vi "BB_CameraMJPG-StreamerRead.vi"(0 "Refnum in":T1, 1 "Operation":enum16{"Read", "Reopen", "Close"}(ring), 2 "remote port or service name":u16=5800, 5 "address":string, 7 "fps":i32=30, 9 "millisecond timer value in":u32, 11 "error in (no error)":errorcluster, 12 "Numeric in":i32) -> (4 "Refnum out":T1, 6 "Numeric 3":i32, 8 "Numeric out":i32, 10 "millisecond timer value out":u32, 15 "error out":errorcluster)   [LabVIEW 2015]
uses:
  <vilib>/vision/Image Controls.llb/IMAQ Image.ctl
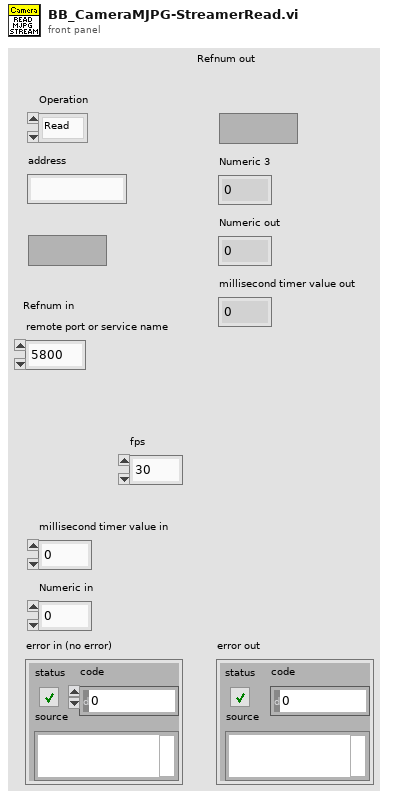
[diagram p1: front panel]
types:
  T1 = typedef "IMAQ Image.ctl" = refnum<image>
  T2 = enum16{"Standard", "Buffered", "CRLF", "Immediate"}
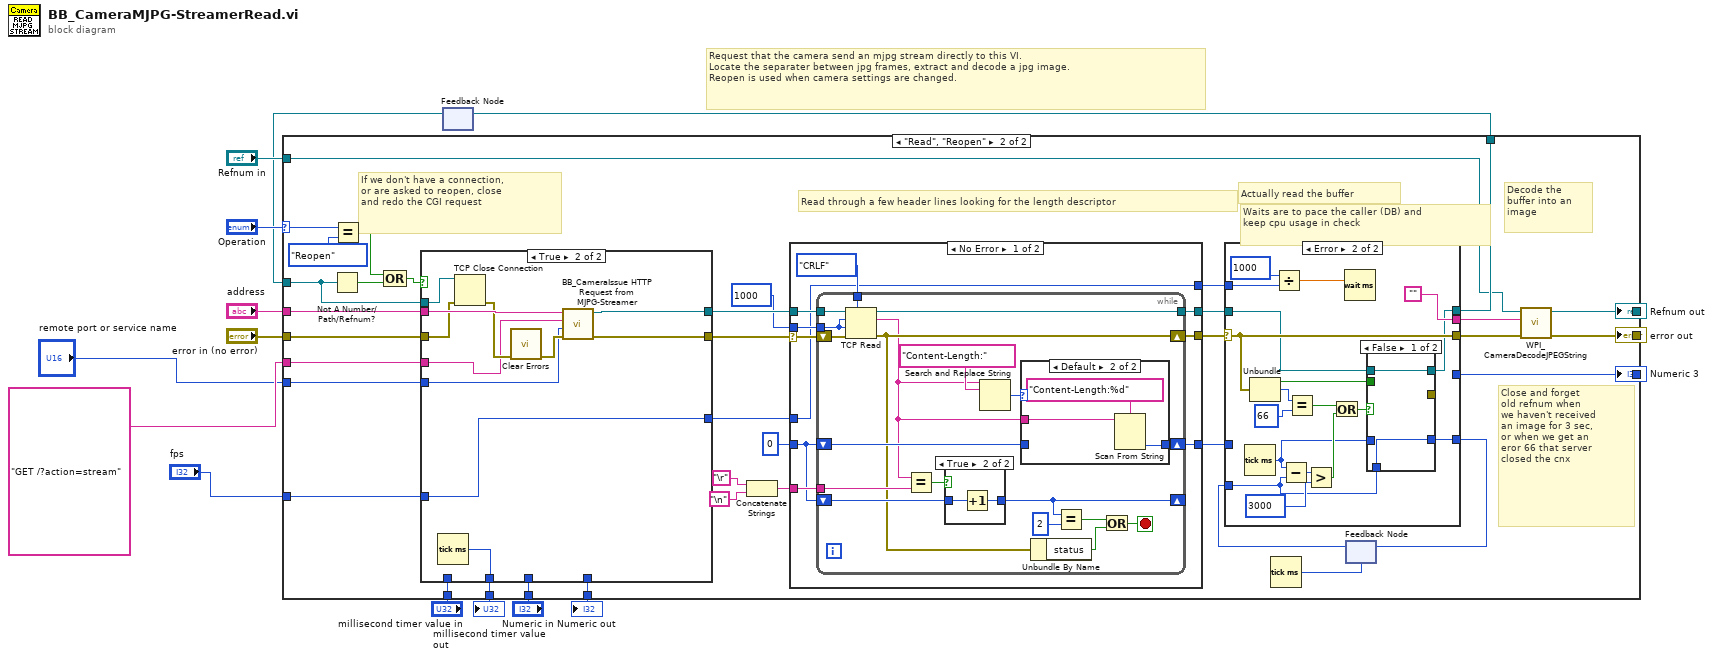
[diagram p0: block diagram]
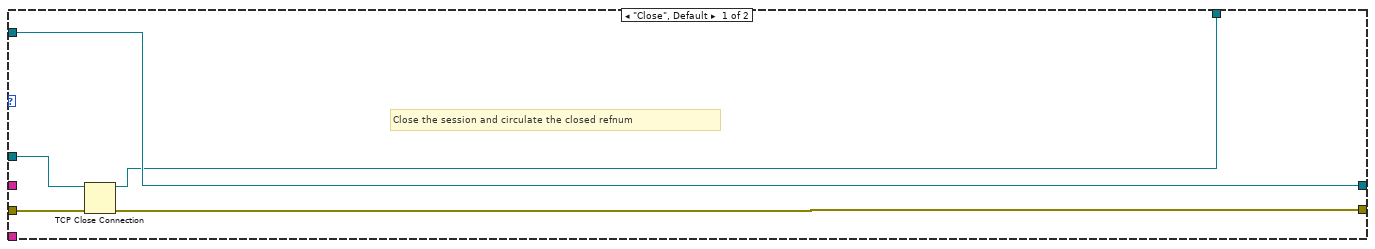
[diagram p2: hidden frame]
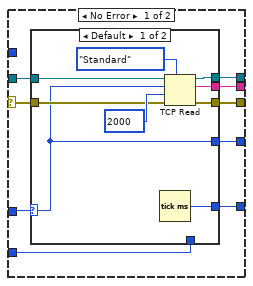
[diagram p4: hidden frame]
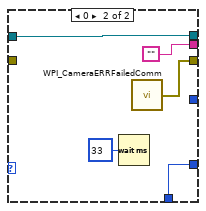
[diagram p5: hidden frame]
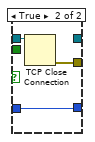
[diagram p6: hidden frame]
diagram:
  # "Request that the camera send an mjpg stream directly to this VI.\nLocate the separater between jpg frames, extract and decode a jpg image.\nReopen is used when camera settings are changed."
  n1 = feedback #1() -> (w9:refnum<k5>)  [unwired: 1 out]
  n2 = case shown="\"Read\", \"Reopen\"" "Operation" {
    selector: "Operation" -> [_ w38]
    tunnel: "error in (no error)" -> [w20 w49]
    tunnel: "address" -> [_ w48]
    tunnel: [w17 w47] -> w6
    tunnel: "GET /?action=stream" -> [_ w46]
    tunnel: [w18 w43] -> w7
    tunnel: [w19 w41] -> w8
    tunnel: w9 -> [w21 w39]
    tunnel: "Refnum in" -> [w18 w37]
    tunnel: [_ w33] -> w12
    tunnel: "Numeric in" -> [_ w32]
    tunnel: [_ w31] -> w14
    tunnel: "millisecond timer value in" -> [_ w30]
    tunnel: [_ w29] -> w16
    tunnel: "fps" -> [_ w23]
    tunnel: "remote port or service name" -> [_ w22]
    frame "Close", Default {
      # "Close the session and circulate the closed refnum"
      n3 = TCP Close Connection(connection ID=w21, error in (no error)=w20) -> (connection ID out=w17:refnum<k5>, error out=w19:errorcluster)  [unwired: 1 out]
    }
    frame "Read", "Reopen" {
      # "Waits are to pace the caller (DB) and\nkeep cpu usage in check"
      # "Close and forget\nold refnum when\nwe haven't received\nan image for 3 sec,\nor when we get an\neror 66 that server\nclosed the cnx"
      # "Decode the buffer into an image"
      # "Actually read the buffer"
      # "Read through a few header lines looking for the length descriptor"
      # "If we don't have a connection,\nor are asked to reopen, close\nand redo the CGI request"
      n4 = Not A Number/Path/Refnum?(number/path/refnum=w39) -> (NaN/Path/Refnum?=w27:bool)
      n5 = Equal?(x=w38, y=enum16{"Read", "Reopen", "Close"}."Reopen" ("Operation")) -> (x = y?=w28:bool)
      n6 = Compound Arithmetic op=OR(w28, w27) -> (w26:bool)
      n7 = case shown="True" w26 {
        tunnel: [w62 w72] -> w53
        tunnel: [w63 w73] -> w52
        tunnel: w49 -> [w62 w70]
        tunnel: w48 -> [_ w74]
        tunnel: w39 -> [w63 w71]
        tunnel: w46 -> [_ w66]
        tunnel: w32 -> [w61 _]
        tunnel: [w61 _] -> w31
        tunnel: w30 -> [w60 _]
        tunnel: [w60 w67] -> w29
        tunnel: [w59 w65] -> w24
        tunnel: w23 -> [w59 w65]
        tunnel: w22 -> [_ w64]
        frame False {
        }
        frame True {
          n8 = Tick Count (ms)() -> (millisecond timer value=w67:u32)
          n9 = TCP Close Connection(connection ID=w71, error in (no error)=w70) -> (error out=w69:errorcluster)  [unwired: 2 out]
          n10 = call <vilib>:"Clear Errors.vi"("error in (no error)"=w69) -> ("error out"=w68:errorcluster)  [unwired: 1 in, 5 out]
          n11 = call "BB_CameraIssue HTTP Request from MJPG-Streamer.vi"("error in (no error)"=w68, "remote port or service name"=w64, "Request"=w66, "address"=w74) -> ("error out"=w72:errorcluster, "connection ID (dup)"=w73:refnum<k5>)  [unwired: 6 out]
        }
      }
      n12 = Concatenate Strings("\r", "\n") -> (w56:string)
      n13 = case shown="No Error" w53 {
        selector: w53 -> [w123 w159]
        tunnel: [w130 w159] -> w50
        tunnel: [w129 w158] -> w55
        tunnel: [w128 w160] -> w54
        tunnel: w56 -> [w127 _]
        tunnel: w52 -> [w125 w160]
        tunnel: 1000 ("bytes to read") -> [w124 _]
        tunnel: 0 -> [w122 w158]
        tunnel: [w121 w157] -> w25
        tunnel: w24 -> [w121 w157]
        frame No Error {
          n14 = while {
            tunnel: w125 -> [w149]
            tunnel: [w148] -> w128
            shift-right: [w147] -> w129
            shift-left: w122 -> [w146]
            shift-right: [w143] -> _
            shift-left: w122 -> [w144]
            tunnel: w127 -> [w141]
            tunnel: w124 -> [w131]
            tunnel: T2."CRLF" ("mode (standard)") -> [w140]
            shift-right: [w138] -> w130
            shift-left: w123 -> [w139]
            stop <- w137 stop-if-true
            n15 = TCP Read(connection ID=w149, bytes to read=w131, error in (no error)=w139, 7:w140, 9:w131) -> (connection ID out=w148:refnum<k5>, data out=w132:string, error out=w138:errorcluster)
            n16 = Equal?(x=w132, y=w141) -> (x = y?=w145:bool)
            n17 = case shown="True" w145 {
              tunnel: w144 -> [w150 w152]
              tunnel: [w150 w151] -> w143
              frame False {
              }
              frame True {
                n18 = Increment(x=w152) -> (x+1=w151:i32)
              }
            }
            n19 = Search and Replace String(input string=w132, search string="Content-Length:" ("regular expression")) -> (number of replacements=w136:i32)  [unwired: 1 in, 8 out]
            n20 = case shown="Default" w136 {
              tunnel: [w153 w156] -> w147
              tunnel: w146 -> [w153 _]
              tunnel: w132 -> [_ w155]
              frame 0 {
              }
              frame Default {
                n21 = Scan From String(format string="Content-Length:%d" ("regular expression"), input string=w155) -> (output 1=w156:i32)  [unwired: 2 in, 4 out]
              }
            }
            n22 = Unbundle By Name(w138) -> ("status"=w133:bool)
            n23 = Equal?(x=w143, y=2) -> (x = y?=w134:bool)
            n24 = Or(x=w134, y=w133) -> (x .or. y?=w137:bool)
          }
        }
        frame Error {
        }
      }
      n25 = Tick Count (ms)() -> (millisecond timer value=w35:u32)
      n26 = feedback #2(w35) -> (w34:u32)
      n27 = case shown="Error" w50 {
        selector: w50 -> [w79 w114]
        tunnel: [w83 w114] -> w42
        tunnel: [w82 ""] -> w44
        tunnel: [w81 w111] -> w47
        tunnel: w55 -> [w78 _]
        tunnel: w54 -> [w80 w112]
        tunnel: [w77 w103] -> w36
        tunnel: w34 -> [w76 w101]
        tunnel: [w75 _] -> w33
        tunnel: w25 -> [_ w98]
        frame No Error {
          n28 = case shown="Default" w78 {
            selector: w78 -> [w84 _]
            tunnel: w80 -> [w92 w96]
            tunnel: [w91 w95] -> w83
            tunnel: [w88 ""] -> w82
            tunnel: [w87 w96] -> w81
            tunnel: w79 -> [w86 _]
            tunnel: [w85 w93] -> w77
            tunnel: w76 -> [_ w93]
            tunnel: [w84 _] -> w75
            frame Default {
              n29 = Tick Count (ms)() -> (millisecond timer value=w85:u32)
              n30 = TCP Read(connection ID=w92, bytes to read=w84, error in (no error)=w86, 7:T2."Standard" ("mode (standard)"), 9:2000 ("timeout ms (25000)")) -> (connection ID out=w87:refnum<k5>, data out=w88:string, error out=w91:errorcluster)
            }
            frame 0 {
              n31 = Wait (ms)(milliseconds to wait=u32 33) -> ()  [unwired: 1 out]
              n32 = call <vilib>:"WPI_CameraERRFailedComm.vi"() -> ("error out"=w95:errorcluster)
            }
          }
        }
        frame Error {
          n33 = Tick Count (ms)() -> (millisecond timer value=w102:u32)
          n34 = Unbundle(w114) -> ("status"=w113:bool, "code"=w109:i32)  [unwired: 1 out]
          n35 = Divide(x=u32 1000 ("milliseconds to wait"), y=w98) -> (x/y=w99:dbl)
          n36 = Subtract(x=w102, y=w101) -> (x-y=w104:u32)
          n37 = Equal?(x=w109, y=u32 66 ("milliseconds to wait")) -> (x = y?=w108:bool)
          n38 = Greater?(x=w104, y=u32 3000 ("milliseconds to wait")) -> (0:w106:bool)
          n39 = Or(x=w108, y=w106) -> (x .or. y?=w107:bool)
          n40 = Wait (ms)(milliseconds to wait=w99) -> ()  [unwired: 1 out]
          n41 = case shown="False" w107 {
            tunnel: w113 -> [_ _]
            tunnel: w112 -> [w117 w120]
            tunnel: [w117 _] -> w111
            tunnel: [w116 w119] -> w103
            tunnel: w102 -> [_ w119]
            tunnel: w101 -> [w116 _]
            tunnel: [_ w118] -> _
            frame False {
            }
            frame True {
              n42 = TCP Close Connection(connection ID=w120) -> (error out=w118:errorcluster)  [unwired: 1 in, 2 out]
            }
          }
        }
      }
      n43 = feedback-in #2(w36) -> ()
      n44 = call <vilib>:"WPI_CameraDecodeJPEGString.vi"("error in"=w42, "Compressed Image"=w44, "Image In"=w37) -> ("error out"=w41:errorcluster, "Image Out"=w43:T1)  [unwired: 3 out]
    }
  }
  "millisecond timer value out" <- w16
  "Numeric out" <- w14
  "Numeric 3" <- w12
  "error out" <- w8
  "Refnum out" <- w7
  n45 = feedback-in #1(w6) -> ()
